vi "Program DUT.vi"(9 "Programming Complete Event":refnum<user-event>, 10 "Position":u32, 11 "Programmer":refnum<class "Programmer.lvclass">) -> ()   [LabVIEW 2015, in "Program RF.lvclass"]
uses:
  Program RF.lvclass
  Classes/Programmer/Programmer/Class/Programmer.lvclass
  <vilib>/Cree, Inc/Cree Test Framework/Classes/Base Objects/Base Class/Base Class/Base Class.lvclass
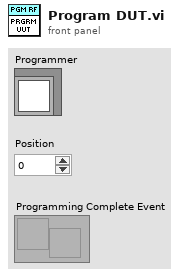
[diagram p1: front panel]
types:
  T1 = cluster{"status":bool, "code":i32, "source":string, "Position":u32}
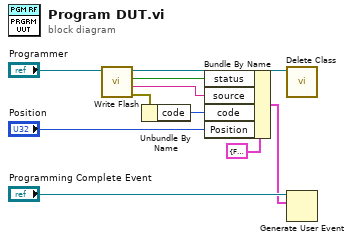
[diagram p0: block diagram]
diagram:
  n1 = call-dynamic "Write Flash.vi"("Acrobat Template in"="Programmer") -> ("error out"=w6:errorcluster, "Response"=w7:string, "Success"=w8:bool, "Acrobat Template out"=w3:refnum<class "Programmer.lvclass">)  [unwired: 7 in]
  n2 = Unbundle By Name(w6) -> ("code"=w5:i32)
  n3 = Bundle By Name(cluster=T1 {"status"=FALSE, "code"=0, "source"="", "Position"=0} ("error IO"), "status"=w8, "source"=w7, "code"=w5, "Position"="Position") -> (w1:T1)
  n4 = call <vilib>:"Delete Class.vi"("Base Class in"=w3) -> ()  [unwired: 9 in, 2 out]
  n5 = Generate User Event(user event="Programming Complete Event", event data cluster=w1) -> ()  [unwired: 2 in, 2 out]
